vi "test_read-nmea-data2.vi"() -> ()   [LabVIEW 2019] (continued)
122,12,85,70,065,21,86,36,330,,3*79\n\t\n15:10:30.59\tF9P\t$GAGSV,2,1,08,02,09,298,08,04,66,119,22,09,31,193,18,11,71,357,24,7*7D\n\t\n15:10:30.61\tF9P\t$GAGSV,2,2,08,12,40,102,11,19,27,045,23,25,09,249,,36,25,308,13,7*78\n\t\n15:10:30.63\tF9P\t$GAGSV,2,1,08,02,09,298,,04,66,119,,09,31,193,16,11,71,357,,2*78\n\t\n15:10:30.65\tF9P\t$GAGSV,2,2,08,12,40,102,,19,27,045,,25,09,249,,36,25,308,,2*7E\n\t\n15:10:30.67\tF9P\t$GBGSV,1,1,03,11,50,131,19,14,87,138,20,33,60,219,22,1*45\n\t\n15:10:30.69\tF9P\t$GBGSV,1,1,03,11,50,131,,14,87,138,21,33,60,219,,3*4E\n\t\n15:10:30.71\tF9P\t$GNGLL,3723.56746,N,12656.88501,E,061032.00,A,A*70\n\t\n15:10:30.73\tF9P\t\t\n15:10:30.75\tF9P\t\t\n15:10:30.77\tF9P\t\t\n15:10:30.79\tF9P\t\t\n15:10:30.81\tF9P\t\t\n15:10:30.83\tF9P\t\t\n15:10:30.85\tF9P\t\t\n15:10:30.87\tF9P\t\t\n15:10:30.89\tF9P\t\t\n15:10:30.91\tF9P\t\t\n15:10:30.93\tF9P\t\t\n15:10:30.95\tF9P\t\t\n15:10:30.97\tF9P\t\t\n15:10:30.99\tF9P\t\t\n15:10:31.01\tF9P\t\t\n15:10:31.03\tF9P\t\t\n15:10:31.05\tF9P\t\t\n15:10:31.07\tF9P\t\t\n15:10:31.09\tF9P\t\t\n15:10:31.11\tF9P\t\t\n15:10:31.13\tF9P\t\t\n15:10:31.15\tF9P\t\t\n15:10:31.17\tF9P\t\t\n15:10:31.19\tF9P\t\t\n15:10:31.21\tF9P\t\t\n15:10:31.23\tF9P\t\t\n15:10:31.25\tF9P\t$GNRMC,061033.00,A,3723.56706,N,12656.88487,E,1.563,,250720,,,A,V*1A\n\t\n15:10:31.27\tF9P\t$GNVTG,,T,,M,1.563,N,2.894,K,A*3B\n\t\n15:10:31.29\tF9P\t$GNGGA,061033.00,3723.56706,N,12656.88487,E,1,12,0.64,62.8,M,18.5,M,,*7E\n\t\n15:10:31.31\tF9P\t$GNGSA,A,3,12,06,19,05,17,09,04,02,,,,,1.18,0.64,1.00,1*0B\n\t\n15:10:31.33\tF9P\t$GNGSA,A,3,85,71,84,,,,,,,,,,1.18,0.64,1.00,2*0E\n\t\n15:10:31.35\tF9P\t$GNGSA,A,3,36,19,11,04,09,12,,,,,,,1.18,0.64,1.00,3*0B\n\t\n15:10:31.37\tF9P\t$GNGSA,A,3,14,11,33,,,,,,,,,,1.18,0.64,1.00,4*0A\n\t\n15:10:31.39\tF9P\t$GPGSV,3,1,09,02,54,318,23,04,18,044,27,05,37,247,22,06,64,047,28,1*62\n\t\n15:10:31.41\tF9P\t$GPGSV,3,2,09,09,45,075,20,12,24,278,17,17,34,153,23,19,53,156,24,1*67\n\t\n15:10:31.43\tF9P\t$GPGSV,3,3,09,25,12,307,08,1*55\n\t\n15:10:31.45\tF9P\t$GPGSV,3,1,09,02,54,318,,04,18,044,,05,37,247,15,06,64,047,14,6*6A\n\t\n15:10:31.47\tF9P\t$GPGSV,3,2,09,09,45,075,13,12,24,278,,17,34,153,16,19,53,156,,6*66\n\t\n15:10:31.49\tF9P\t$GPGSV,3,3,09,25,12,307,,6*5A\n\t\n15:10:31.51\tF9P\t$GLGSV,2,1,08,69,12,031,,70,72,041,,71,51,205,16,72,03,209,,1*75\n\t\n15:10:31.53\tF9P\t$GLGSV,2,2,08,77,01,326,,84,20,122,09,85,70,065,20,86,36,330,,1*70\n\t\n15:10:31.55\tF9P\t$GLGSV,2,1,08,69,12,031,,70,72,041,,71,51,205,18,72,03,209,,3*79\n\t\n15:10:31.57\tF9P\t$GLGSV,2,2,08,77,01,326,,84,20,122,09,85,70,065,19,86,36,330,,3*78\n\t\n15:10:31.59\tF9P\t$GAGSV,2,1,08,02,09,298,07,04,66,119,22,09,31,193,16,11,71,357,24,7*7C\n\t\n15:10:31.61\tF9P\t$GAGSV,2,2,08,12,40,102,10,19,27,045,25,25,09,249,,36,25,308,13,7*7F\n\t\n15:10:31.63\tF9P\t$GAGSV,2,1,08,02,09,298,,04,66,119,,09,31,193,16,11,71,357,,2*78\n\t\n15:10:31.65\tF9P\t$GAGSV,2,2,08,12,40,102,,19,27,045,,25,09,249,,36,25,308,,2*7E\n\t\n15:10:31.67\tF9P\t$GBGSV,1,1,03,11,50,131,22,14,87,138,21,33,60,219,20,1*4E\n\t\n15:10:31.69\tF9P\t$GBGSV,1,1,03,11,50,131,29,14,87,138,21,33,60,219,,3*45\n\t\n15:10:31.71\tF9P\t$GNGLL,3723.56706,N,12656.88487,E,061033.00,A,A*7A\n\t\n15:10:31.73\tF9P\t\t\n15:10:31.75\tF9P\t\t\n15:10:31.77\tF9P\t\t\n15:10:31.79\tF9P\t\t\n15:10:31.81\tF9P\t\t\n15:10:31.83\tF9P\t\t\n15:10:31.85\tF9P\t\t\n15:10:31.87\tF9P\t\t\n15:10:31.89\tF9P\t\t\n15:10:31.91\tF9P\t\t\n15:10:31.93\tF9P\t\t\n15:10:31.95\tF9P\t\t\n15:10:31.97\tF9P\t\t\n15:10:31.99\tF9P\t\t\n15:10:32.01\tF9P\t\t\n15:10:32.03\tF9P\t\t\n15:10:32.05\tF9P\t\t\n15:10:32.07\tF9P\t\t\n15:10:32.09\tF9P\t\t\n15:10:32.11\tF9P\t\t\n15:10:32.13\tF9P\t\t\n15:10:32.15\tF9P\t\t\n15:10:32.17\tF9P\t\t\n15:10:32.19\tF9P\t\t\n15:10:32.21\tF9P\t\t\n15:10:32.23\tF9P\t\t\n15:10:32.25\tF9P\t$GNRMC,061034.00,A,3723.56670,N,12656.88505,E,1.096,,250720,,,A,V*19\n\t\n15:10:32.27\tF9P\t$GNVTG,,T,,M,1.096,N,2.030,K,A*32\n\t\n15:10:32.29\tF9P\t$GNGGA,061034.00,3723.56670,N,12656.88505,E,1,12,0.64,63.4,M,18.5,M,,*7F\n\t\n15:10:32.31\tF9P\t$GNGSA,A,3,12,06,19,05,17,09,04,02,,,,,1.18,0.64,1.00,1*0B\n\t\n15:10:32.33\tF9P\t$GNGSA,A,3,85,71,84,,,,,,,,,,1.18,0.64,1.00,2*0E\n\t\n15:10:32.35\tF9P\t$GNGSA,A,3,36,19,11,04,09,12,,,,,,,1.18,0.64,1.00,3*0B\n\t\n15:10:32.37\tF9P\t$GNGSA,A,3,14,11,33,,,,,,,,,,1.18,0.64,1.00,4*0A\n\t\n15:10:32.39\tF9P\t$GPGSV,3,1,09,02,54,318,23,04,18,044,26,05,37,247,22,06,64,047,27,1*6C\n\t\n15:10:32.41\tF9P\t$GPGSV,3,2,09,09,45,075,20,12,24,278,16,17,34,153,25,19,53,156,24,1*60\n\t\n15:10:32.43\tF9P\t$GPGSV,3,3,09,25,12,307,09,1*54\n\t\n15:10:32.45\tF9P\t$GPGSV,3,1,09,02,54,318,,04,18,044,,05,37,247,15,06,64,047,13,6*6D\n\t\n15:10:32.47\tF9P\t$GPGSV,3,2,09,09,45,075,12,12,24,278,,17,34,153,15,19,53,156,,6*64\n\t\n15:10:32.49\tF9P\t$GPGSV,3,3,09,25,12,307,,6*5A\n\t\n15:10:32.51\tF9P\t$GLGSV,2,1,08,69,12,031,,70,72,041,,71,51,205,15,72,03,209,,1*76\n\t\n15:10:32.53\tF9P\t$GLGSV,2,2,08,77,01,326,,84,20,122,10,85,70,065,19,86,36,330,,1*72\n\t\n15:10:32.55\tF9P\t$GLGSV,2,1,08,69,12,031,,70,72,041,,71,51,205,17,72,03,209,,3*76\n\t\n15:10:32.57\tF9P\t$GLGSV,2,2,08,77,01,326,,84,20,122,11,85,70,065,18,86,36,330,,3*70\n\t\n15:10:32.59\tF9P\t$GAGSV,2,1,08,02,09,298,09,04,66,119,22,09,31,193,17,11,71,357,23,7*74\n\t\n15:10:32.61\tF9P\t$GAGSV,2,2,08,12,40,102,11,19,27,045,24,25,09,249,,36,25,308,13,7*7F\n\t\n15:10:32.63\tF9P\t$GAGSV,2,1,08,02,09,298,,04,66,119,,09,31,193,16,11,71,357,,2*78\n\t\n15:10:32.65\tF9P\t$GAGSV,2,2,08,12,40,102,,19,27,045,,25,09,249,,36,25,308,,2*7E\n\t\n15:10:32.67\tF9P\t$GBGSV,1,1,03,11,50,131,22,14,87,138,21,33,60,219,19,1*44\n\t\n15:10:32.69\tF9P\t$GBGSV,1,1,03,11,50,131,28,14,87,138,21,33,60,219,,3*44\n\t\n15:10:32.71\tF9P\t$GNGLL,3723.56670,N,12656.88505,E,061034.00,A,A*76\n\t\n15:10:32.73\tF9P\t\t\n15:10:32.75\tF9P\t\t\n15:10:32.77\tF9P\t\t\n15:10:32.79\tF9P\t\t\n15:10:32.81\tF9P\t\t\n15:10:32.83\tF9P\t\t\n15:10:32.85\tF9P\t\t\n15:10:32.87\tF9P\t\t\n15:10:32.89\tF9P\t\t\n15:10:32.91\tF9P\t\t\n15:10:32.93\tF9P\t\t\n15:10:32.95\tF9P\t\t\n15:10:32.97\tF9P\t\t\n15:10:32.99\tF9P\t\t\n15:10:33.01\tF9P\t\t\n15:10:33.03\tF9P\t\t\n15:10:33.05\tF9P\t\t\n15:10:33.07\tF9P\t\t\n15:10:33.09\tF9P\t\t\n15:10:33.11\tF9P\t\t\n15:10:33.13\tF9P\t\t\n15:10:33.15\tF9P\t\t\n15:10:33.17\tF9P\t\t\n15:10:33.19\tF9P\t\t\n15:10:33.21\tF9P\t\t\n15:10:33.23\tF9P\t\t\n15:10:33.25\tF9P\t$GNRMC,061035.00,A,3723.56608,N,12656.88519,E,1.607,,250720,,,A,V*14\n\t\n15:10:33.27\tF9P\t$GNVTG,,T,,M,1.607,N,2.976,K,A*37\n\t\n15:10:33.29\tF9P\t$GNGGA,061035.00,3723.56608,N,12656.88519,E,1,12,0.64,63.9,M,18.5,M,,*71\n\t\n15:10:33.31\tF9P\t$GNGSA,A,3,12,06,19,05,17,09,04,02,,,,,1.18,0.64,1.00,1*0B\n\t\n15:10:33.33\tF9P\t$GNGSA,A,3,85,71,84,,,,,,,,,,1.18,0.64,1.00,2*0E\n\t\n15:10:33.35\tF9P\t$GNGSA,A,3,36,19,11,04,09,12,,,,,,,1.18,0.64,1.00,3*0B\n\t\n15:10:33.37\tF9P\t$GNGSA,A,3,14,11,33,,,,,,,,,,1.18,0.64,1.00,4*0A\n\t\n15:10:33.39\tF9P\t$GPGSV,3,1,09,02,54,318,23,04,18,044,25,05,37,247,29,06,64,047,26,1*65\n\t\n15:10:33.41\tF9P\t$GPGSV,3,2,09,09,45,074,20,12,24,278,17,17,34,153,24,19,53,156,22,1*67\n\t\n15:10:33.43\tF9P\t$GPGSV,3,3,09,25,12,307,12,1*5E\n\t\n15:10:33.45\tF9P\t$GPGSV,3,1,09,02,54,318,,04,18,044,,05,37,247,16,06,64,047,14,6*69\n\t\n15:10:33.47\tF9P\t$GPGSV,3,2,09,09,45,074,11,12,24,278,,17,34,153,15,19,53,156,,6*66\n\t\n15:10:33.49\tF9P\t$GPGSV,3,3,09,25,12,307,,6*5A\n\t\n15:10:33.51\tF9P\t$GLGSV,2,1,08,69,12,031,,70,72,041,,71,51,205,16,72,03,209,,1*75\n\t\n15:10:33.53\tF9P\t$GLGSV,2,2,08,77,01,326,,84,20,122,08,85,70,065,20,86,36,330,,1*71\n\t\n15:10:33.55\tF9P\t$GLGSV,2,1,08,69,12,031,,70,72,041,,71,51,205,16,72,03,209,,3*77\n\t\n15:10:33.57\tF9P\t$GLGSV,2,2,08,77,01,326,,84,20,122,12,85,70,065,19,86,36,330,,3*72\n\t\n15:10:33.59\tF9P\t$GAGSV,2,1,08,02,09,298,08,04,66,119,24,09,31,193,19,11,71,357,23,7*7D\n\t\n15:10:33.61\tF9P\t$GAGSV,2,2,08,12,40,102,10,19,27,045,24,25,09,249,,36,25,308,11,7*7C\n\t\n15:10:33.63\tF9P\t$GAGSV,2,1,08,02,09,298,,04,66,119,,09,31,193,18,11,71,357,,2*76\n\t\n15:10:33.65\tF9P\t$GAGSV,2,2,08,12,40,102,,19,27,045,,25,09,249,,36,25,308,,2*7E\n\t\n15:10:33.67\tF9P\t$GBGSV,1,1,03,11,50,131,22,14,87,138,19,33,60,219,19,1*4F\n\t\n15:10:33.69\tF9P\t$GBGSV,1,1,03,11,50,131,28,14,87,138,21,33,60,219,,3*44\n\t\n15:10:33.71\tF9P\t$GNGLL,3723.56608,N,12656.88519,E,061035.00,A,A*75\n\t\n15:10:33.73\tF9P\t\t\n15:10:33.75\tF9P\t\t\n15:10:33.77\tF9P\t\t\n15:10:33.79\tF9P\t\t\n15:10:33.81\tF9P\t\t\n15:10:33.83\tF9P\t\t\n15:10:33.85\tF9P\t\t\n15:10:33.87\tF9P\t\t\n15:10:33.89\tF9P\t\t\n15:10:33.91\tF9P\t\t\n15:10:33.93\tF9P\t\t\n15:10:33.95\tF9P\t\t\n15:10:33.97\tF9P\t\t\n15:10:33.99\tF9P\t\t\n15:10:34.01\tF9P\t\t\n15:10:34.03\tF9P\t\t\n15:10:34.05\tF9P\t\t\n15:10:34.07\tF9P\t\t\n15:10:34.09\tF9P\t\t\n15:10:34.11\tF9P\t\t\n15:10:34.13\tF9P\t\t\n15:10:34.15\tF9P\t\t\n15:10:34.17\tF9P\t\t\n15:10:34.19\tF9P\t\t\n15:10:34.21\tF9P\t\t\n15:10:34.23\tF9P\t\t\n15:10:34.25\tF9P\t$GNRMC,061036.00,A,3723.56564,N,12656.88522,E,1.240,,250720,,,A,V*11\n\t\n15:10:34.27\tF9P\t$GNVTG,,T,,M,1.240,N,2.297,K,A*34\n\t\n15:10:34.29\tF9P\t$GNGGA,061036.00,3723.56564,N,12656.88522,E,1,12,0.64,63.8,M,18.5,M,,*72\n\t\n15:10:34.31\tF9P\t$GNGSA,A,3,12,06,19,05,17,09,04,02,,,,,1.18,0.64,1.00,1*0B\n\t\n15:10:34.33\tF9P\t$GNGSA,A,3,85,71,84,,,,,,,,,,1.18,0.64,1.00,2*0E\n\t\n15:10:34.35\tF9P\t$GNGSA,A,3,36,19,11,04,09,12,,,,,,,1.18,0.64,1.00,3*0B\n\t\n15:10:34.37\tF9P\t$GNGSA,A,3,14,11,33,,,,,,,,,,1.18,0.64,1.00,4*0A\n\t\n15:10:34.39\tF9P\t$GPGSV,3,1,09,02,54,318,23,04,18,044,25,05,37,247,25,06,64,047,25,1*6A\n\t\n15:10:34.41\tF9P\t$GPGSV,3,2,09,09,45,074,19,12,24,278,19,17,34,153,24,19,53,156,22,1*63\n\t\n15:10:34.43\tF9P\t$GPGSV,3,3,09,25,12,307,13,1*5F\n\t\n15:10:34.45\tF9P\t$GPGSV,3,1,09,02,54,318,,04,18,044,,05,37,247,16,06,64,047,14,6*69\n\t\n15:10:34.47\tF9P\t$GPGSV,3,2,09,09,45,074,11,12,24,278,,17,34,153,16,19,53,156,,6*65\n\t\n15:10:34.49\tF9P\t$GPGSV,3,3,09,25,12,307,,6*5A\n\t\n15:10:34.51\tF9P\t$GLGSV,2,1,08,69,12,031,,70,72,041,,71,51,205,17,72,03,209,,1*74\n\t\n15:10:34.53\tF9P\t$GLGSV,2,2,08,77,01,326,,84,20,122,08,85,70,065,22,86,36,330,,1*73\n\t\n15:10:34.55\tF9P\t$GLGSV,2,1,08,69,12,031,,70,72,041,,71,51,205,19,72,03,209,,3*78\n\t\n15:10:34.57\tF9P\t$GLGSV,2,2,08,77,01,326,,84,20,122,10,85,70,065,19,86,36,330,,3*70\n\t\n15:10:34.59\tF9P\t$GAGSV,2,1,08,02,09,298,08,04,66,119,25,09,31,193,19,11,71,357,23,7*7C\n\t\n15:10:34.61\tF9P\t$GAGSV,2,2,08,12,40,102,13,19,27,045,30,25,09,249,,36,25,308,10,7*7B\n\t\n15:10:34.63\tF9P\t$GAGSV,2,1,08,02,09,298,,04,66,119,,09,31,193,18,11,71,357,,2*76\n\t\n15:10:34.65\tF9P\t$GAGSV,2,2,08,12,40,102,,19,27,045,,25,09,249,,36,25,308,,2*7E\n\t\n15:10:34.67\tF9P\t$GBGSV,1,1,03,11,50,131,21,14,87,138,19,33,60,219,19,1*4C\n\t\n15:10:34.69\tF9P\t$GBGSV,1,1,03,11,50,131,21,14,87,138,22,33,60,219,,3*4E\n\t\n15:10:34.71\tF9P\t$GNGLL,3723.56564,N,12656.88522,E,061036.00,A,A*77\n\t\n15:10:34.73\tF9P\t\t\n15:10:34.75\tF9P\t\t\n15:10:34.77\tF9P\t\t\n15:10:34.79\tF9P\t\t\n15:10:34.81\tF9P\t\t\n15:10:34.83\tF9P\t\t\n15:10:34.85\tF9P\t\t\n15:10:34.87\tF9P\t\t\n15:10:34.89\tF9P\t\t\n15:10:34.91\tF9P\t\t\n15:10:34.93\tF9P\t\t\n15:10:34.95\tF9P\t\t\n15:10:34.97\tF9P\t\t\n15:10:34.99\tF9P\t\t\n15:10:35.01\tF9P\t\t\n15:10:35.03\tF9P\t\t\n15:10:35.05\tF9P\t\t\n15:10:35.07\tF9P\t\t\n15:10:35.09\tF9P\t\t\n15:10:35.11\tF9P\t\t\n15:10:35.13\tF9P\t\t\n15:10:35.15\tF9P\t\t\n15:10:35.17\tF9P\t\t\n15:10:35.19\tF9P\t\t\n15:10:35.21\tF9P\t\t\n15:10:35.23\tF9P\t\t\n15:10:35.25\tF9P\t$GNRMC,061037.00,A,3723.56478,N,12656.88570,E,3.100,159.41,250720,,,A,V*08\n\t\n15:10:35.27\tF9P\t$GNVTG,159.41,T,,M,3.100,N,5.741,K,A*2E\n\t\n15:10:35.29\tF9P\t$GNGGA,061037.00,3723.56478,N,12656.88570,E,1,12,0.64,63.9,M,18.5,M,,*79\n\t\n15:10:35.31\tF9P\t$GNGSA,A,3,12,06,19,05,17,09,04,02,,,,,1.18,0.64,1.00,1*0B\n\t\n15:10:35.33\tF9P\t$GNGSA,A,3,85,71,84,,,,,,,,,,1.18,0.64,1.00,2*0E\n\t\n15:10:35.35\tF9P\t$GNGSA,A,3,36,19,11,04,09,12,,,,,,,1.18,0.64,1.00,3*0B\n\t\n15:10:35.37\tF9P\t$GNGSA,A,3,14,11,33,,,,,,,,,,1.18,0.64,1.00,4*0A\n\t\n15:10:35.39\tF9P\t$GPGSV,3,1,09,02,54,318,23,04,18,044,25,05,37,247,25,06,64,047,26,1*69\n\t\n15:10:35.41\tF9P\t$GPGSV,3,2,09,09,45,074,19,12,24,278,21,17,34,153,24,19,53,156,23,1*69\n\t\n15:10:35.43\tF9P\t$GPGSV,3,3,09,25,12,307,15,1*59\n\t\n15:10:35.45\tF9P\t$GPGSV,3,1,09,02,54,318,,04,18,044,,05,37,247,15,06,64,047,15,6*6B\n\t\n15:10:35.47\tF9P\t$GPGSV,3,2,09,09,45,074,,12,24,278,,17,34,153,15,19,53,156,,6*66\n\t\n15:10:35.49\tF9P\t$GPGSV,3,3,09,25,12,307,,6*5A\n\t\n15:10:35.51\tF9P\t$GLGSV,2,1,08,69,12,031,,70,72,041,,71,51,205,17,72,03,209,,1*74\n\t\n15:10:35.53\tF9P\t$GLGSV,2,2,08,77,01,326,,84,20,122,10,85,70,065,21,86,36,330,,1*79\n\t\n15:10:35.55\tF9P\t$GLGSV,2,1,08,69,12,031,,70,72,041,,71,51,205,18,72,03,209,,3*79\n\t\n15:10:35.57\tF9P\t$GLGSV,2,2,08,77,01,326,,84,20,122,08,85,70,065,17,86,36,330,,3*77\n\t\n15:10:35.59\tF9P\t$GAGSV,2,1,08,02,09,298,11,04,66,119,25,09,31,193,20,11,71,357,26,7*7B\n\t\n15:10:35.61\tF9P\t$GAGSV,2,2,08,12,40,102,09,19,27,045,24,25,09,249,,36,25,308,09,7*7D\n\t\n15:10:35.63\tF9P\t$GAGSV,2,1,08,02,09,298,,04,66,119,,09,31,193,17,11,71,357,,2*79\n\t\n15:10:35.65\tF9P\t$GAGSV,2,2,08,12,40,102,,19,27,045,,25,09,249,,36,25,308,,2*7E\n\t\n15:10:35.67\tF9P\t$GBGSV,1,1,03,11,50,131,21,14,87,138,16,33,60,219,20,1*49\n\t\n15:10:35.69\tF9P\t$GBGSV,1,1,03,11,50,131,29,14,87,138,22,33,60,219,,3*46\n\t\n15:10:35.71\tF9P\t$GNGLL,3723.56478,N,12656.88570,E,061037.00,A,A*7D\n\t\n15:10:35.73\tF9P\t\t\n15:10:35.75\tF9P\t\t\n15:10:35.77\tF9P\t\t\n15:10:35.79\tF9P\t\t\n15:10:35.81\tF9P\t\t\n15:10:35.83\tF9P\t\t\n15:10:35.85\tF9P\t\t\n15:10:35.87\tF9P\t\t\n15:10:35.89\tF9P\t\t\n15:10:35.91\tF9P\t\t\n15:10:35.93\tF9P\t\t\n15:10:35.95\tF9P\t\t\n15:10:35.97\tF9P\t\t\n15:10:35.99\tF9P\t\t\n15:10:36.01\tF9P\t\t\n15:10:36.03\tF9P\t\t\n15:10:36.05\tF9P\t\t\n15:10:36.07\tF9P\t\t\n15:10:36.09\tF9P\t\t\n15:10:36.11\tF9P\t\t\n15:10:36.13\tF9P\t\t\n15:10:36.15\tF9P\t\t\n15:10:36.17\tF9P\t\t\n15:10:36.19\tF9P\t\t\n15:10:36.21\tF9P\t\t\n15:10:36.23\tF9P\t\t\n15:10:36.25\tF9P\t$GNRMC,061038.00,A,3723.56429,N,12656.88590,E,1.510,,250720,,,A,V*1C\n\t\n15:10:36.27\tF9P\t$GNVTG,,T,,M,1.510,N,2.797,K,A*33\n\t\n15:10:36.29\tF9P\t$GNGGA,061038.00,3723.56429,N,12656.88590,E,1,12,0.64,64.6,M,18.5,M,,*74\n\t\n15:10:36.31\tF9P\t$GNGSA,A,3,12,06,19,05,17,09,04,02,,,,,1.18,0.64,1.00,1*0B\n\t\n15:10:36.33\tF9P\t$GNGSA,A,3,85,71,84,,,,,,,,,,1.18,0.64,1.00,2*0E\n\t\n15:10:36.35\tF9P\t$GNGSA,A,3,36,19,11,04,09,12,,,,,,,1.18,0.64,1.00,3*0B\n\t\n15:10:36.37\tF9P\t$GNGSA,A,3,14,11,33,,,,,,,,,,1.18,0.64,1.00,4*0A\n\t\n15:10:36.39\tF9P\t$GPGSV,3,1,09,02,54,318,29,04,18,044,25,05,37,247,25,06,64,047,27,1*62\n\t\n15:10:36.41\tF9P\t$GPGSV,3,2,09,09,45,074,18,12,24,277,23,17,34,153,24,19,53,156,22,1*64\n\t\n15:10:36.43\tF9P\t$GPGSV,3,3,09,25,12,307,18,1*54\n\t\n15:10:36.45\tF9P\t$GPGSV,3,1,09,02,54,318,,04,18,044,,05,37,247,14,06,64,047,16,6*69\n\t\n15:10:36.47\tF9P\t$GPGSV,3,2,09,09,45,074,,12,24,277,,17,34,153,18,19,53,156,,6*64\n\t\n15:10:36.49\tF9P\t$GPGSV,3,3,09,25,12,307,,6*5A\n\t\n15:10:36.51\tF9P\t$GLGSV,2,1,08,69,12,031,,70,72,041,,71,51,205,17,72,03,209,,1*74\n\t\n15:10:36.53\tF9P\t$GLGSV,2,2,08,77,01,326,,84,20,122,08,85,70,065,20,86,36,330,,1*71\n\t\n15:10:36.55\tF9P\t$GLGSV,2,1,08,69,12,031,,70,72,041,,71,51,205,19,72,03,209,,3*78\n\t\n15:10:36.57\tF9P\t$GLGSV,2,2,08,77,01,326,,84,20,122,08,85,70,065,20,86,36,330,,3*73\n\t\n15:10:36.59\tF9P\t$GAGSV,2,1,08,02,09,298,08,04,66,119,25,09,31,193,20,11,71,357,27,7*72\n\t\n15:10:36.61\tF9P\t$GAGSV,2,2,08,12,40,102,10,19,27,045,24,25,09,249,,36,25,308,10,7*7D\n\t\n15:10:36.63\tF9P\t$GAGSV,2,1,08,02,09,298,,04,66,119,,09,31,193,19,11,71,357,,2*77\n\t\n15:10:36.65\tF9P\t$GAGSV,2,2,08,12,40,102,,19,27,045,,25,09,249,,36,25,308,,2*7E\n\t\n15:10:36.67\tF9P\t$GBGSV,1,1,03,11,50,131,21,14,87,138,17,33,60,219,21,1*49\n\t\n15:10:36.69\tF9P\t$GBGSV,1,1,03,11,50,131,,14,87,138,22,33,60,219,,3*4D\n\t\n15:10:36.71\tF9P\t$GNGLL,3723.56429,N,12656.88590,E,061038.00,A,A*78\n\t\n15:10:36.73\tF9P\t\t\n15:10:36.75\tF9P\t\t\n15:10:36.77\tF9P\t\t\n15:10:36.79\tF9P\t\t\n15:10:36.81\tF9P\t\t\n15:10:36.83\tF9P\t\t\n15:10:36.85\tF9P\t\t\n15:10:36.87\tF9P\t\t\n15:10:36.89\tF9P\t\t\n15:10:36.91\tF9P\t\t\n15:10:36.93\tF9P\t\t\n15:10:36.95\tF9P\t\t\n15:10:36.97\tF9P\t\t\n15:10:36.99\tF9P\t\t\n15:10:37.01\tF9P\t\t\n15:10:37.03\tF9P\t\t\n15:10:37.05\tF9P\t\t\n15:10:37.07\tF9P\t\t\n15:10:37.09\tF9P\t\t\n15:10:37.11\tF9P\t\t\n15:10:37.13\tF9P\t\t\n15:10:37.15\tF9P\t\t\n15:10:37.17\tF9P\t\t\n15:10:37.19\tF9P\t\t\n15:10:37.21\tF9P\t\t\n15:10:37.23\tF9P\t\t\n15:10:37.25\tF9P\t$GNRMC,061039.00,A,3723.56378,N,12656.88565,E,1.969,,250720,,,A,V*16\n\t\n15:10:37.27\tF9P\t$GNVTG,,T,,M,1.969,N,3.647,K,A*3C\n\t\n15:10:37.29\tF9P\t$GNGGA,061039.00,3723.56378,N,12656.88565,E,1,12,0.64,64.4,M,18.5,M,,*7E\n\t\n15:10:37.31\tF9P\t$GNGSA,A,3,12,06,19,05,17,09,04,02,,,,,1.18,0.64,1.00,1*0B\n\t\n15:10:37.33\tF9P\t$GNGSA,A,3,85,71,84,,,,,,,,,,1.18,0.64,1.00,2*0E\n\t\n15:10:37.35\tF9P\t$GNGSA,A,3,36,19,11,04,09,12,,,,,,,1.18,0.64,1.00,3*0B\n\t\n15:10:37.37\tF9P\t$GNGSA,A,3,14,11,33,,,,,,,,,,1.18,0.64,1.00,4*0A\n\t\n15:10:37.39\tF9P\t$GPGSV,3,1,09,02,54,318,24,04,18,044,25,05,37,247,24,06,64,047,26,1*6F\n\t\n15:10:37.41\tF9P\t$GPGSV,3,2,09,09,45,074,20,12,24,277,24,17,34,153,24,19,53,156,22,1*68\n\t\n15:10:37.43\tF9P\t$GPGSV,3,3,09,25,12,307,20,1*5F\n\t\n15:10:37.45\tF9P\t$GPGSV,3,1,09,02,54,318,,04,18,044,,05,37,247,12,06,64,047,16,6*6F\n\t\n15:10:37.47\tF9P\t$GPGSV,3,2,09,09,45,074,,12,24,277,,17,34,153,17,19,53,156,,6*6B\n\t\n15:10:37.49\tF9P\t$GPGSV,3,3,09,25,12,307,,6*5A\n\t\n15:10:37.51\tF9P\t$GLGSV,2,1,08,69,12,031,,70,72,041,,71,51,205,18,72,03,209,,1*7B\n\t\n15:10:37.53\tF9P\t$GLGSV,2,2,08,77,01,326,,84,20,122,10,85,70,065,22,86,36,330,,1*7A\n\t\n15:10:37.55\tF9P\t$GLGSV,2,1,08,69,12,031,,70,72,041,,71,51,205,19,72,03,209,,3*78\n\t\n15:10:37.57\tF9P\t$GLGSV,2,2,08,77,01,326,,84,20,122,11,85,70,065,20,86,36,330,,3*7B\n\t\n15:10:37.59\tF9P\t$GAGSV,2,1,08,02,09,298,06,04,66,119,24,09,31,193,20,11,71,357,25,7*7F\n\t\n15:10:37.61\tF9P\t$GAGSV,2,2,08,12,40,102,11,19,27,045,23,25,09,249,,36,25,308,14,7*7F\n\t\n15:10:37.63\tF9P\t$GAGSV,2,1,08,02,09,298,,04,66,119,,09,31,193,,11,71,357,,2*7F\n\t\n15:10:37.65\tF9P\t$GAGSV,2,2,08,12,40,102,,19,27,045,,25,09,249,,36,25,308,,2*7E\n\t\n15:10:37.67\tF9P\t$GBGSV,1,1,03,11,50,131,22,14,87,138,17,33,60,219,20,1*4B\n\t\n15:10:37.69\tF9P\t$GBGSV,1,1,03,11,50,131,26,14,87,138,22,33,60,219,,3*49\n\t\n15:10:37.71\tF9P\t$GNGLL,3723.56378,N,12656.88565,E,061039.00,A,A*70\n\t\n15:10:37.73\tF9P\t\t\n15:10:37.75\tF9P\t\t\n15:10:37.77\tF9P\t\t\n15:10:37.79\tF9P\t\t\n15:10:37.81\tF9P\t\t\n15:10:37.83\tF9P\t\t\n15:10:37.85\tF9P\t\t\n15:10:37.87\tF9P\t\t\n15:10:37.89\tF9P\t\t\n15:10:37.91\tF9P\t\t\n15:10:37.93\tF9P\t\t\n15:10:37.95\tF9P\t\t\n15:10:37.97\tF9P\t\t\n15:10:37.99\tF9P\t\t\n15:10:38.01\tF9P\t\t\n15:10:38.03\tF9P\t\t\n15:10:38.05\tF9P\t\t\n15:10:38.07\tF9P\t\t\n15:10:38.09\tF9P\t\t\n15:10:38.11\tF9P\t\t\n15:10:38.13\tF9P\t\t\n15:10:38.15\tF9P\t\t\n15:10:38.17\tF9P\t\t\n15:10:38.19\tF9P\t\t\n15:10:38.21\tF9P\t\t\n15:10:38.23\tF9P\t\t\n15:10:38.25\tF9P\t$GNRMC,061040.00,A,3723.56308,N,12656.88574,E,1.884,163.16,250720,,,A,V*00\n\t\n15:10:38.27\tF9P\t$GNVTG,163.16,T,,M,1.884,N,3.489,K,A*23\n\t\n15:10:38.29\tF9P\t$GNGGA,061040.00,3723.56308,N,12656.88574,E,1,12,0.67,64.8,M,18.5,M,,*78\n\t\n15:10:38.31\tF9P\t$GNGSA,A,3,12,06,19,05,17,09,04,02,,,,,1.20,0.67,1.00,1*03\n\t\n15:10:38.33\tF9P\t$GNGSA,A,3,85,71,84,,,,,,,,,,1.20,0.67,1.00,2*06\n\t\n15:10:38.35\tF9P\t$GNGSA,A,3,36,19,11,04,09,12,,,,,,,1.20,0.67,1.00,3*03\n\t\n15:10:38.37\tF9P\t$GNGSA,A,3,14,11,33,,,,,,,,,,1.20,0.67,1.00,4*02\n\t\n15:10:38.39\tF9P\t$GPGSV,3,1,09,02,54,318,24,04,18,044,31,05,37,247,31,06,64,047,32,1*6B\n\t\n15:10:38.41\tF9P\t$GPGSV,3,2,09,09,45,074,20,12,24,277,25,17,34,153,25,19,53,156,30,1*6B\n\t\n15:10:38.43\tF9P\t$GPGSV,3,3,09,25,12,307,19,1*55\n\t\n15:10:38.45\tF9P\t$GPGSV,3,1,09,02,54,318,,04,18,044,,05,37,247,,06,64,047,17,6*6D\n\t\n15:10:38.47\tF9P\t$GPGSV,3,2,09,09,45,074,,12,24,277,,17,34,153,18,19,
